vi "Post-Build Action_NoUICopy.vi"(4 "measurement plugin service":refnum<class "Measurement Plugin Service.lvclass">, 5 "Files Generated by Build":path[](array[path]), 6 "Top Level/Always Included VIs":path[](array[path]), 7 "Destination Path":path, 8 "error in (no error)":errorcluster, 9 "Target Name":string, 10 "Build Specification Name":string, 11 "Project Path":path) -> (0 "error out":errorcluster)   [LabVIEW 2021]
uses:
  <vilib>/Utility/config.llb/Write Key (String).vi
  <vilib>/ErrorRing/Error Ring.xnode
  <vilib>/MeasurementLink/MeasurementLink Measurement Server/Measurement Plugin Service/Measurement Plugin Service.lvclass
  <vilib>/Utility/config.llb/NI_LVConfig.lvlib
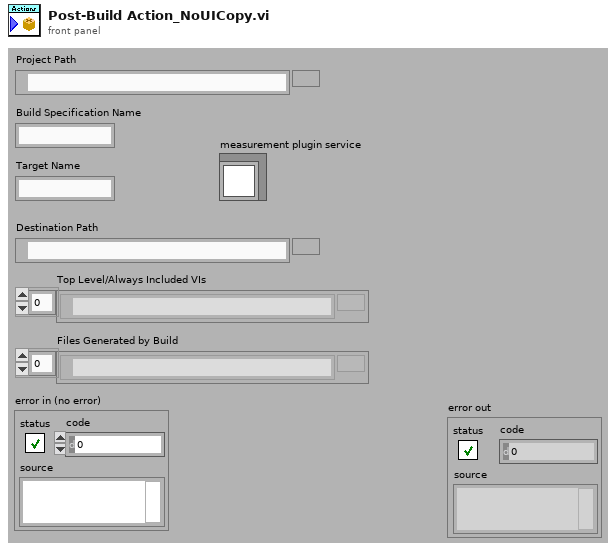
[diagram p1: front panel]
types:
  T1 = cluster{"Target Name":string, "Top Level/Always Included VIs":path[], "Project Path":path, "Destination Path":path, "Build Specification Name":string, "Files Generated by Build":path[]}
  T2 = cluster{"displayName":string, "serviceClass":string, "providedInterfaces":string[], "path":string, "descriptionUrl":string}
  T3 = cluster{"services":cluster{"displayName":string, "serviceClass":string, "providedInterfaces":string[], "path":string, "descriptionUrl":string}[]}
  T4 = typedef "MeasurementLink Measurement Server.lvlib/User Interface Details.ctl" = cluster{"file url":string}
  T5 = typedef "MeasurementLink Measurement Server.lvlib/Measurement Details.ctl" = cluster{"display name":string, "version":string}
  T6 = cluster{"displayName":string, "serviceClass":string, "providedInterfaces":string[], "path":string, "descriptionUrl":string}[]
  T7 = typedef "NI_LVConfig.lvlib/Config Data RefNum.ctl" = refnum<k1>
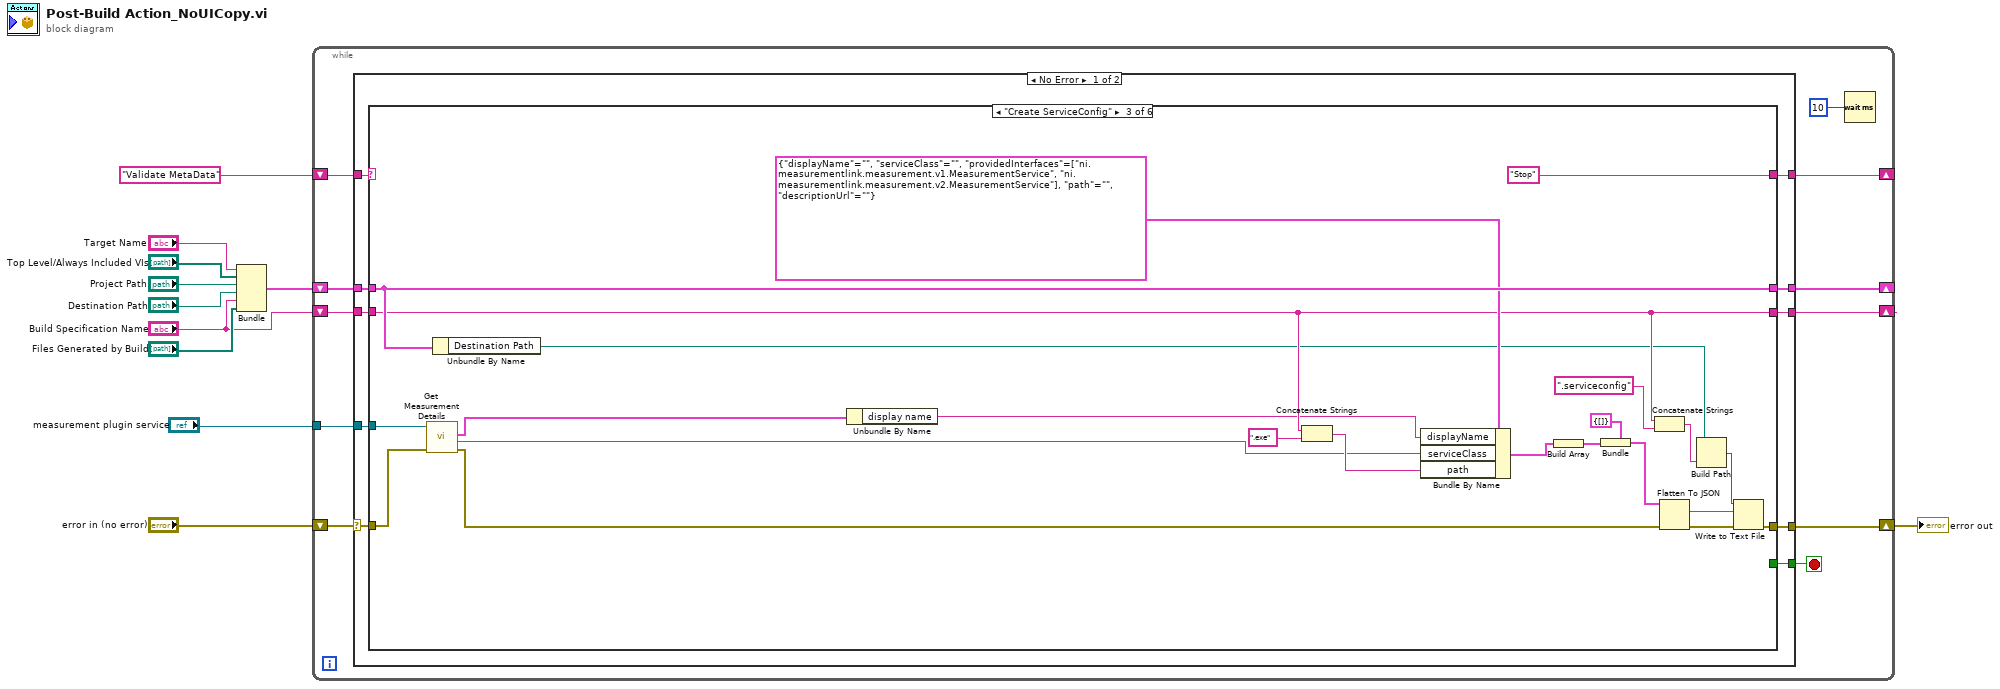
[diagram p0: block diagram]
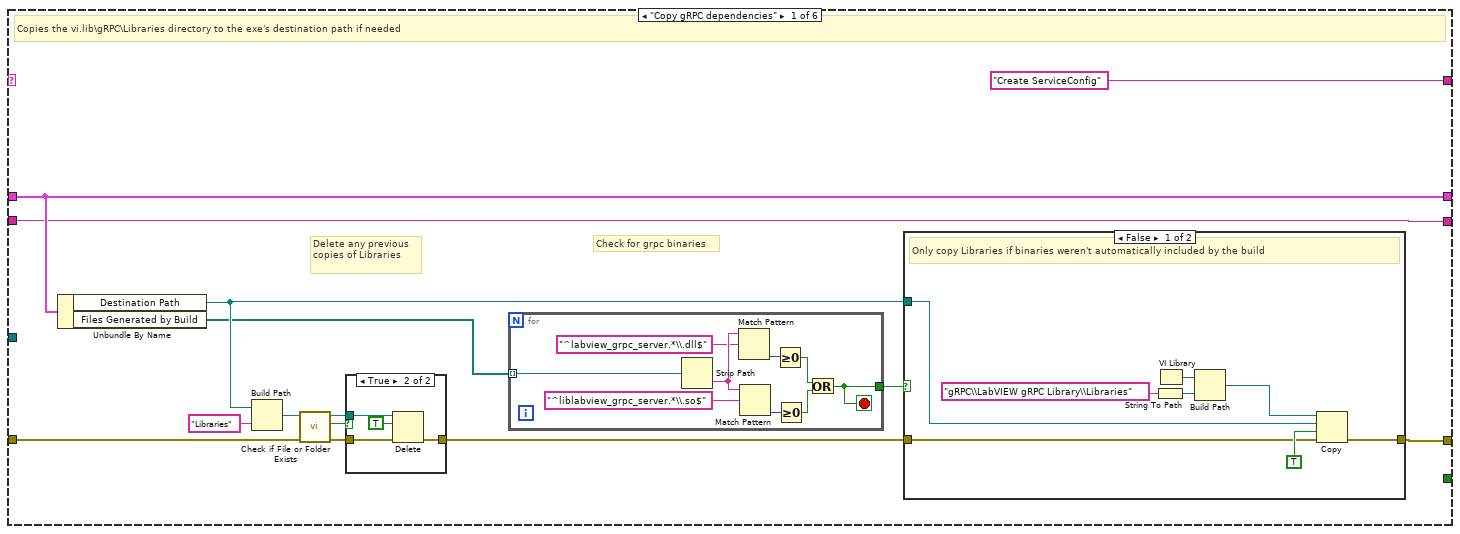
[diagram p2: hidden frame]
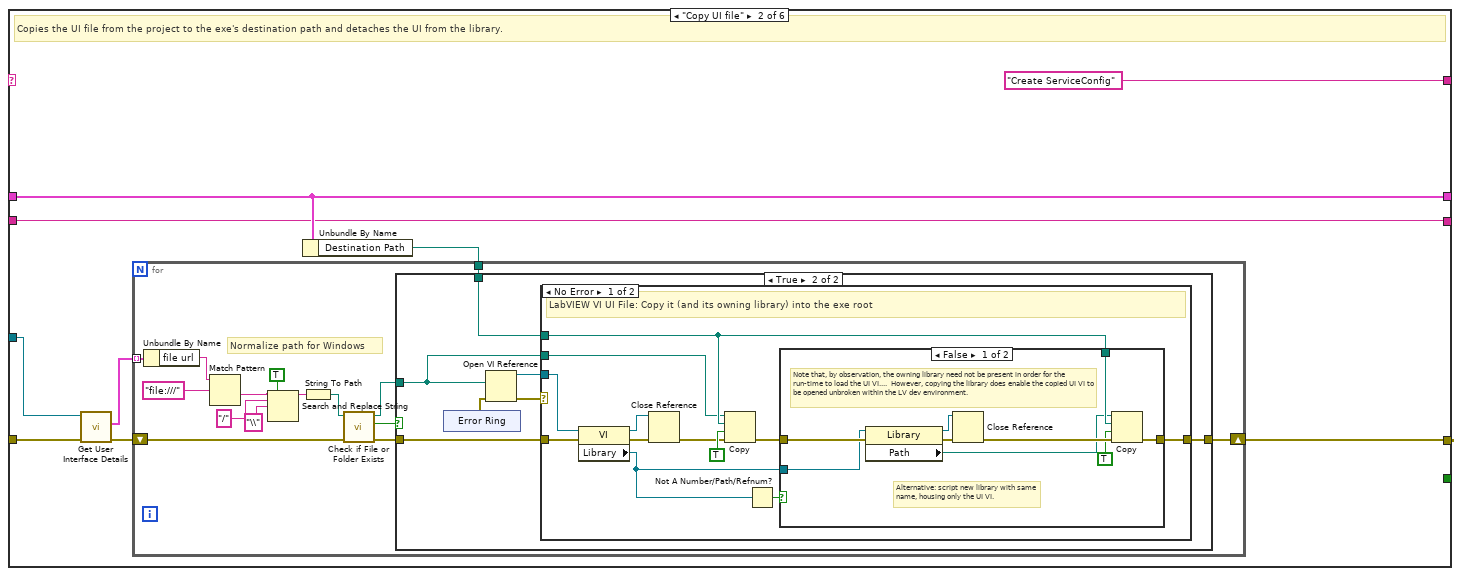
[diagram p5: hidden frame]
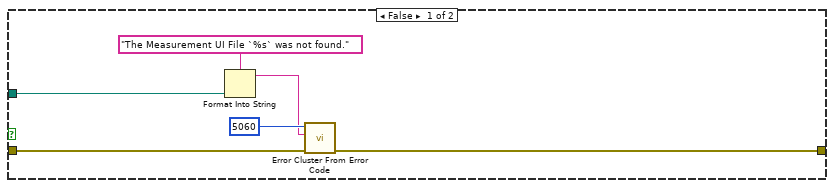
[diagram p6: hidden frame]
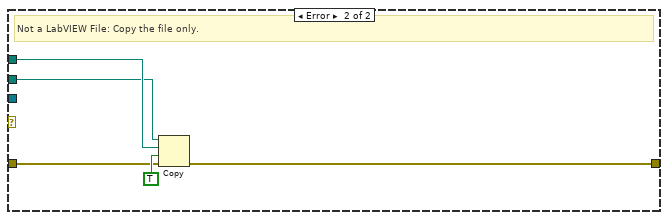
[diagram p8: hidden frame]
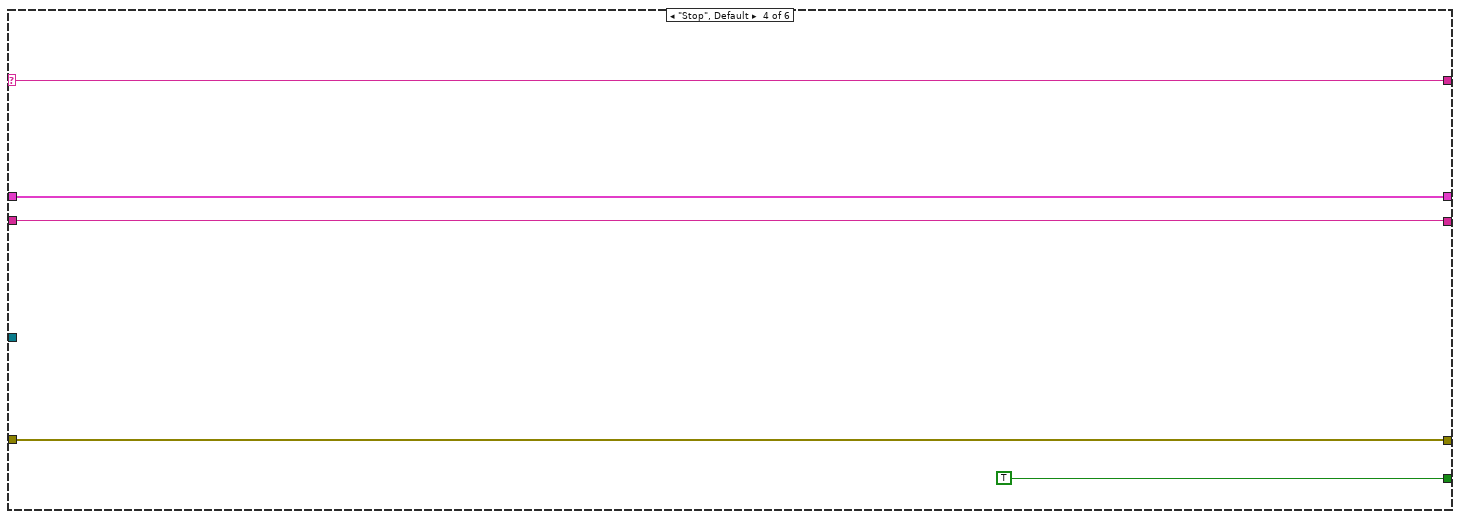
[diagram p9: hidden frame]
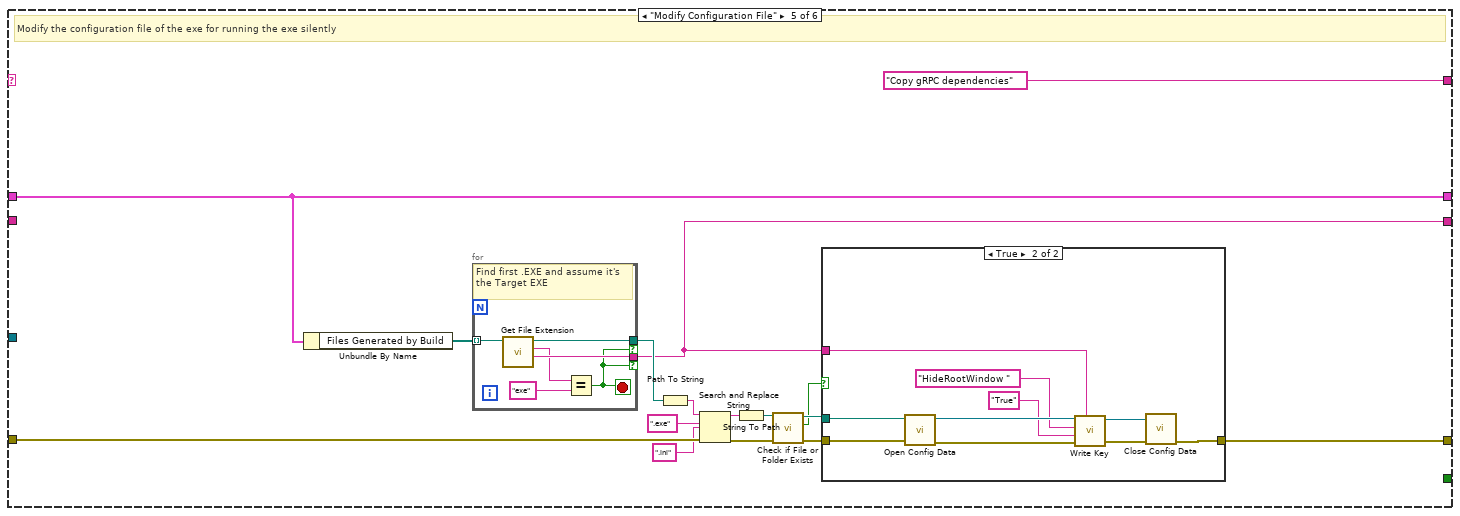
[diagram p10: hidden frame]
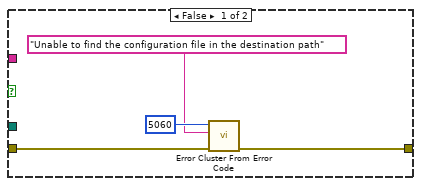
[diagram p11: hidden frame]
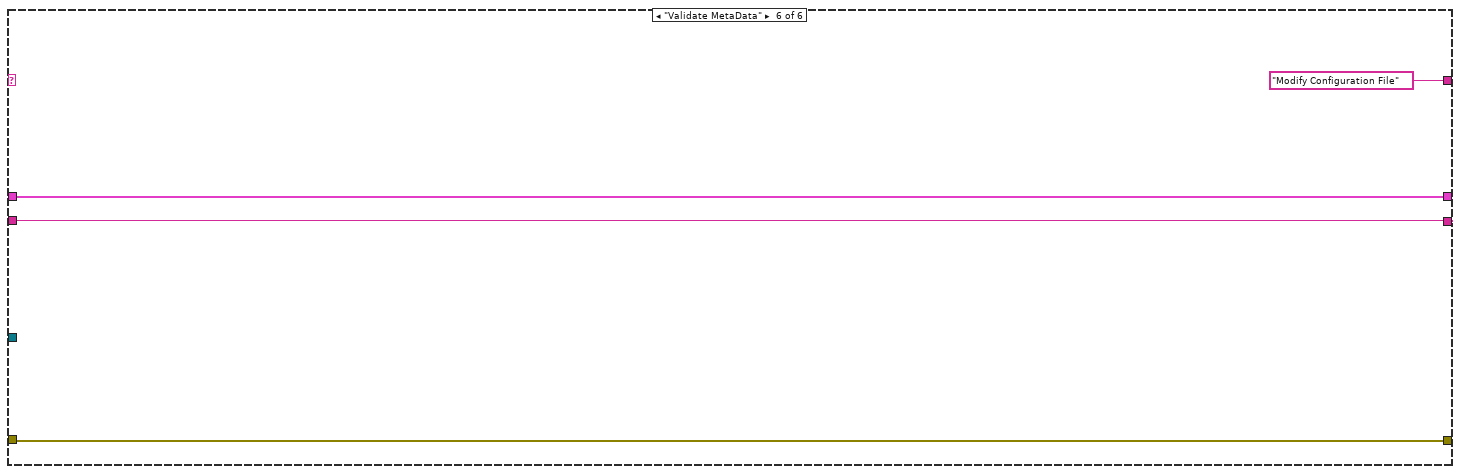
[diagram p12: hidden frame]
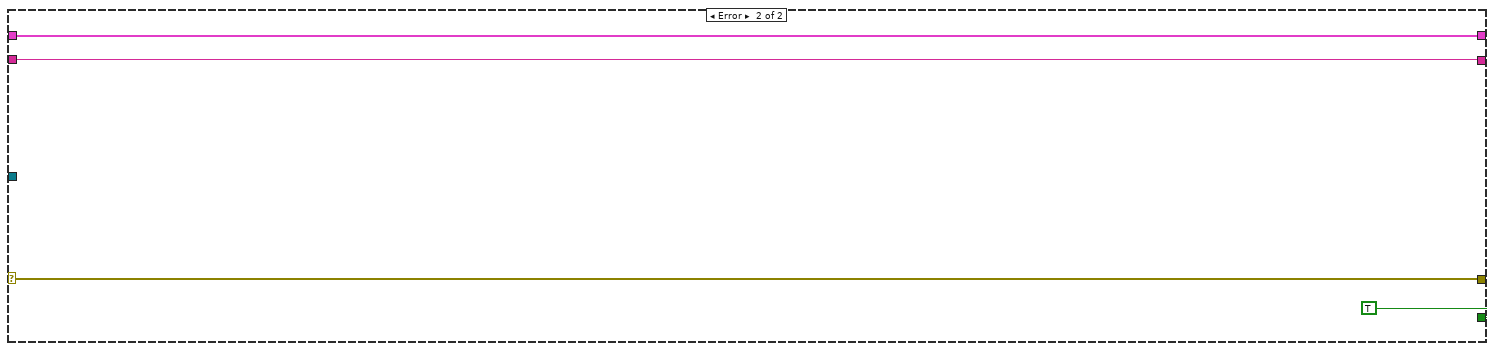
[diagram p13: hidden frame]
diagram:
  n1 = Bundle("Target Name"="Target Name", "Top Level/Always Included VIs"="Top Level/Always Included VIs", "Project Path"="Project Path", "Destination Path"="Destination Path", "Build Specification Name"="Build Specification Name", "Files Generated by Build"="Files Generated by Build") -> (w5:T1)  [unwired: 1 in]
  n2 = while {
    shift-right: [w19] -> _
    shift-left: w5 -> [w20]
    shift-right: [w18] -> w3
    shift-left: "error in (no error)" -> [w15]
    shift-right: [w17] -> _
    shift-left: "Validate MetaData" -> [w21]
    shift-right: [w14] -> _
    shift-left: "Build Specification Name" -> [w13]
    tunnel: "measurement plugin service" -> [w12]
    stop <- w16 stop-if-true
    n3 = case shown="No Error" w15 {
      selector: w15 -> [w26 w205]
      tunnel: w21 -> [w32 _]
      tunnel: w20 -> [w31 w206]
      tunnel: [w30 w206] -> w19
      tunnel: [w29 w205] -> w18
      tunnel: [w28 _] -> w17
      tunnel: [w27 TRUE] -> w16
      tunnel: [w25 w203] -> w14
      tunnel: w13 -> [w24 w203]
      tunnel: w12 -> [w23 _]
      frame No Error {
        n4 = case shown="\"Create ServiceConfig\"" w32 {
          selector: w32 -> [_ _ _ w160 _ _]
          tunnel: w31 -> [w44 w78 w157 w162 w174 w201]
          tunnel: [w44 w78 w157 w162 w174 w201] -> w30
          tunnel: w26 -> [w36 w73 w139 w159 w172 w202]
          tunnel: [w46 w77 w143 w159 w178 w202] -> w29
          tunnel: ["Create ServiceConfig" "Create ServiceConfig" "Stop" w160 "Copy gRPC dependencies" "Modify Configuration File"] -> w28
          tunnel: [_ _ _ TRUE _ _] -> w27
          tunnel: [w43 w74 w148 w158 w164 w200] -> w25
          tunnel: w24 -> [w43 w74 w148 w158 _ w200]
          tunnel: w23 -> [_ w72 w140 _ _ _]
          frame "Copy gRPC dependencies" {
            # "Delete any previous copies of Libraries"
            # "Check for grpc binaries"
            # "Copies the vi.lib\\gRPC\\Libraries directory to the exe's destination path if needed"
            n5 = Unbundle By Name(w44) -> ("Destination Path"=w35:path, "Files Generated by Build"=w33:path[])
            n6 = Build Path(base path=w35, name or relative path="Libraries") -> (appended path=w41:path)
            n7 = call <vilib>:"Check if File or Folder Exists.vi"("error in (no error)"=w36, "path"=w41) -> ("error out"=w40:errorcluster, "file or folder exists?"=w38:bool, "dup path"=w39:path)  [unwired: 7 in]
            n8 = case shown="True" w38 {
              tunnel: w40 -> [w56 w60]
              tunnel: [w56 w59] -> w34
              tunnel: w39 -> [_ w57]
              frame False {
              }
              frame True {
                n9 = Delete(path (use dialog)=w57, entire hierarchy (F)=TRUE ("confirm (F)"), error in=w60) -> (error out=w59:errorcluster)  [unwired: 2 in, 2 out]
              }
            }
            n10 = for {
              tunnel: [w47] -> w42
              tunnel: w33 -> [w52] mode=indexing
              stop <- w47 stop-if-true
              n11 = Strip Path(path=w52) -> (name=w55:string)  [unwired: 1 out]
              n12 = Match Pattern(string=w55, regular expression="^labview_grpc_server.*\\.dll$" ("pattern")) -> (offset past match=w51:i32)  [unwired: 1 in, 3 out]
              n13 = Match Pattern(string=w55, regular expression="^liblabview_grpc_server.*\\.so$" ("pattern")) -> (offset past match=w50:i32)  [unwired: 1 in, 3 out]
              n14 = Greater Or Equal To 0?(x=w51) -> (x >= 0?=w49:bool)
              n15 = Greater Or Equal To 0?(x=w50) -> (x >= 0?=w48:bool)
              n16 = Or(x=w49, y=w48) -> (x .or. y?=w47:bool)
            }
            n17 = case shown="False" w42 {
              tunnel: [w64 w69] -> w46
              tunnel: w35 -> [w62 _]
              tunnel: w34 -> [w61 w69]
              frame False {
                # "Only copy Libraries if binaries weren't automatically included by the build"
                n18 = String To Path(string="gRPC\\LabVIEW gRPC Library\\Libraries") -> (path=w66:path)
                n19 = VI Library() -> (path=w68:path)
                n20 = Build Path(base path=w68, name or relative path=w66) -> (appended path=w65:path)
                n21 = Copy(8:w61, 9:TRUE ("overwrite (F)"), 10:w62, 11:w65) -> (0:w64:errorcluster)  [unwired: 1 in, 2 out]
              }
              frame True {
              }
            }
          }
          frame "Copy UI file" {
            # "Copies the UI file from the project to the exe's destination path and detaches the UI from the library."
            n22 = call-dynamic "Get User Interface Details.vi"("error in"=w73, "measurement plugin service in"=w72) -> ("error out"=w71:errorcluster, "user interface details"=w70:T4[])  [unwired: 7 in, 1 out]
            n23 = Unbundle By Name(w78) -> ("Destination Path"=w75:path)
            n24 = for {
              tunnel: w75 -> [w89]
              tunnel: w70 -> [w92] mode=indexing
              shift-right: [w93] -> w77
              shift-left: w71 -> [w88]
              # "Normalize path for Windows"
              n25 = Unbundle By Name(w92) -> ("file url"=w90:string)
              n26 = Match Pattern(string=w90, regular expression="file:///") -> (after substring=w83:string)  [unwired: 1 in, 3 out]
              n27 = Search and Replace String(replace all?=TRUE ("replace all? (F)"), input string=w83, search string="/" ("after substring"), replace string="\\" ("after substring")) -> (result string=w82:string)  [unwired: 4 in, 3 out]
              n28 = String To Path(string=w82) -> (path=w86:path)
              n29 = call <vilib>:"Check if File or Folder Exists.vi"("error in (no error)"=w88, "path"=w86) -> ("error out"=w87:errorcluster, "file or folder exists?"=w84:bool, "dup path"=w85:path)  [unwired: 7 in]
              n30 = case shown="True" w84 {
                tunnel: [w97 w106] -> w93
                tunnel: w89 -> [_ w102]
                tunnel: w87 -> [w98 w101]
                tunnel: w85 -> [w95 w100]
                frame False {
                  n31 = Format Into String(format string="The Measurement UI File `%s` was not found." ("error message (\"\")"), w95) -> (resulting string=w94:string)  [unwired: 2 in, 1 out]
                  n32 = call <vilib>:"Error Cluster From Error Code.vi"("error in (no error)"=w98, "error message (\"\")"=w94, "error code (0)"=5060) -> ("error out"=w97:errorcluster)  [unwired: 6 in]
                }
                frame True {
                  n33 = xnode "Error Ring"() -> ("error out"=w105:errorcluster)
                  n34 = Open VI Reference(vi path=w100, error in (no error)=w105) -> (vi reference=w103:refnum<vi>, error out=w104:errorcluster)  [unwired: 4 in]
                  n35 = case shown="No Error" w104 {
                    tunnel: w101 -> [w118 w133]
                    tunnel: [w111 w132] -> w106
                    tunnel: w103 -> [w119 _]
                    tunnel: w102 -> [w115 w131]
                    tunnel: w100 -> [w108 w130]
                    frame No Error {
                      # "LabVIEW VI UI File: Copy it (and its owning library) into the exe root"
                      n36 = property class="VI"(reference=w119, error in=w118) -> (reference out=w117:refnum<vi>, error out=w116:errorcluster, "Library"=w112:refnum<vi>)
                      n37 = Close Reference(reference=w117, error in (no error)=w116) -> (error out=w109:errorcluster)
                      n38 = Copy(8:w109, 9:TRUE ("overwrite (F)"), 10:w115, 11:w108) -> (0:w110:errorcluster)  [unwired: 1 in, 2 out]
                      n39 = Not A Number/Path/Refnum?(number/path/refnum=w112) -> (NaN/Path/Refnum?=w113:bool)
                      n40 = case shown="False" w113 {
                        tunnel: [w127 w129] -> w111
                        tunnel: w115 -> [w125 _]
                        tunnel: w110 -> [w123 w129]
                        tunnel: w112 -> [w122 _]
                        frame False {
                          # "Alternative: script new library with same name, housing only the UI VI."
                          # "Note that, by observation, the owning library need not be present in order for the run-time to load the UI VI....  However, copying the library does enable the copied UI VI to be opened unbroken within the LV dev environment."
                          n41 = property class="Library"(reference=w122, error in=w123) -> (reference out=w121:refnum<vi>, error out=w120:errorcluster, "Path"=w124:path)
                          n42 = Close Reference(reference=w121, error in (no error)=w120) -> (error out=w128:errorcluster)
                          n43 = Copy(8:w128, 9:TRUE ("overwrite (F)"), 10:w125, 11:w124) -> (0:w127:errorcluster)  [unwired: 1 in, 2 out]
                        }
                        frame True {
                        }
                      }
                    }
                    frame Error {
                      # "Not a LabVIEW File: Copy the file only."
                      n44 = Copy(8:w133, 9:TRUE ("overwrite (F)"), 10:w131, 11:w130) -> (0:w132:errorcluster)  [unwired: 1 in, 2 out]
                    }
                  }
                }
              }
            }
          }
          frame "Create ServiceConfig" {
            n45 = call-dynamic "Get Measurement Details.vi"("error in"=w139, "measurement plugin service in"=w140) -> ("error out"=w138:errorcluster, "service class"=w135:string, "measurement details"=w137:T5)  [unwired: 5 in, 2 out]
            n46 = Unbundle By Name(w157) -> ("Destination Path"=w146:path)
            n47 = Unbundle By Name(w137) -> ("display name"=w136:string)
            n48 = Concatenate Strings(w148, ".exe" ("string")) -> (w141:string)
            n49 = Bundle By Name(cluster=T2 {"displayName"="", "serviceClass"="", "providedInterfaces"=["ni.measurementlink.measurement.v1.MeasurementService", "ni.measurementlink.measurement.v2.MeasurementService"], "path"="", "descriptionUrl"=""}, "displayName"=w136, "serviceClass"=w135, "path"=w141) -> (w152:T2)
            n50 = Build Array(w152) -> (w151:T6)
            n51 = Bundle(cluster=T3 {"services"=[]}, "services"=w151) -> (w150:T3)
            n52 = Concatenate Strings(w148, ".serviceconfig" ("string")) -> (w145:string)
            n53 = Flatten To JSON(anything=w150, error in (no error)=w138) -> (JSON string=w149:string, 11:w144:errorcluster)  [unwired: 1 in]
            n54 = Build Path(base path=w146, name or relative path=w145) -> (appended path=w142:path)
            n55 = Write to Text File(file (use dialog)=w142, text=w149, error in=w144) -> (error out=w143:errorcluster)  [unwired: 1 in, 2 out]
          }
          frame "Stop", Default {
          }
          frame "Modify Configuration File" {
            # "Modify the configuration file of the exe for running the exe silently"
            n56 = Unbundle By Name(w174) -> ("Files Generated by Build"=w173:path[])
            n57 = for {
              tunnel: w173 -> [w184] mode=indexing
              tunnel: [w183] -> w164 if=w179
              tunnel: [w182] -> w166 if=w179
              stop <- w179 stop-if-true
              # "Find first .EXE and assume it's the Target EXE"
              n58 = call <vilib>:"Get File Extension.vi"("file"=w184) -> ("filename without extension"=w183:string, "lowercase file extension"=w180:string, "dup file"=w182:path)  [unwired: 6 in, 2 out]
              n59 = Equal?(x=w180, y="exe") -> (x = y?=w179:bool)
            }
            n60 = Path To String(path=w166) -> (string=w165:string)
            n61 = Search and Replace String(input string=w165, search string=".exe", replace string=".ini", error in=w172) -> (result string=w169:string, error out=w171:errorcluster)  [unwired: 4 in, 2 out]
            n62 = String To Path(string=w169) -> (path=w168:path)
            n63 = call <vilib>:"Check if File or Folder Exists.vi"("error in (no error)"=w171, "path"=w168) -> ("error out"=w177:errorcluster, "file or folder exists?"=w175:bool, "dup path"=w176:path)  [unwired: 7 in]
            n64 = case shown="True" w175 {
              tunnel: [w187 w198] -> w178
              tunnel: w176 -> [_ w191]
              tunnel: w177 -> [w188 w190]
              tunnel: w164 -> [_ w189]
              frame False {
                n65 = call <vilib>:"Error Cluster From Error Code.vi"("error in (no error)"=w188, "error message (\"\")"="Unable to find the configuration file in the destination path" ("source"), "error code (0)"=5060) -> ("error out"=w187:errorcluster)  [unwired: 6 in]
              }
              frame True {
                n66 = call <vilib>:"Open Config Data.vi"("error in (no error)"=w190, "configuration file path"=w191) -> ("error out"=w197:errorcluster, "refnum"=w196:T7)  [unwired: 7 in, 1 out]
                n67 = call-poly <vilib>:"Write Key.vi"("section"=w189, "error in (no error)"=w197, "value"="True", "key"="HideRootWindow ", "refnum"=w196) -> ("error out"=w194:errorcluster, "refnum out"=w193:T7)  [unwired: 4 in, 1 out]
                n68 = call <vilib>:"Close Config Data.vi"("error in (no error)"=w194, "refnum"=w193) -> ("error out"=w198:errorcluster)  [unwired: 8 in, 1 out]
              }
            }
          }
          frame "Validate MetaData" {
          }
        }
      }
      frame Error {
      }
    }
    n69 = Wait (ms)(milliseconds to wait=u32 10 ("millisecond timer value")) -> ()  [unwired: 1 out]
  }
  "error out" <- w3
